vi "ModbusRxLoop.vi"(11 "ModbusPortSettings":T1={"TxPort"="ModbusPort1Tx", "TxDataFIFO"="ModbusPort1TxFIFO", "TxInternalDataFIFO"="ModbusPort1TxInternalFIFO", "TxHealthAndStatusFIFO"="ModbusPort1TxHealthAndStatusFIFO", "RxPort"="ModbusPort1Rx", "RxDataFIFO"="ModbusPort1RxFIFO", "RxHealthAndStatusFIFO"="ModbusPort1RxHealthAndStatusFIFO", "WaitForRxFrameRegister"="ModbusPort1WaitForRxControl", "BaseHealthAndStatusAddress"=0, "IRQAddress"=0, "TriggerIRQRegister"="ModbusPort1IRQControl", "SoftwareControlledTrigger"="ModbusSoftwareControlledTrigger", "TimestampRegister"="TimestampRegister", "TxTimestampFIFO"="ModbusPort1TimestampFIFO"}) -> ()   [LabVIEW 2016, in "FPGAModbus.lvlib"]
uses:
  FPGAModbus.lvlib
  DataTypes/ModbusPortSettings.ctl
  DataTypes/ModbusRxLoopData.ctl
  DataTypes/ModbusRxStates.ctl
  <vilib>/Platform/TimedLoop/XDataNode/timing_clust.ctl
  <vilib>/Platform/TimedLoop/XDataNode/nitl_modes.ctl
  <vilib>/Platform/TimedLoop/XDataNode/wakeup.ctl
  Common_FPGA_HealthAndStatus/DataTypes/HealthAndStatusUpdateMode.ctl
  <vilib>/rvi/Emulation/niFpgaSctlEmulationGetInTimedLoop.vi
  <vilib>/rvi/Emulation/niFpgaEmulationReportErrorSimple.vi
  <vilib>/rvi/Emulation/niFpgaGetClockAttributes.vi
  <vilib>/rvi/Emulation/niFpgaCriticalErrorInLSC.vi
  <vilib>/rvi/DataTransferAndStorage/Container/Common/niFpgaContainerExecOnDevCompGetState.vi
  <vilib>/rvi/Emulation/niFpgaEmulationIsFPGAContextNoSignature.vi
  <vilib>/rvi/DataTransferAndStorage/Container/Common/niFpgaContainerGetUniqueNameForEmu.vi
  <vilib>/rvi/Memory/Memory_Emulation/niFpgaMemoryEmulationCacheClearOnFirstRun.vi
  <vilib>/rvi/Memory/Memory_Emulation/nirvimemoryEmulationManagerCache_MakeExclusive.vi
  <vilib>/rvi/Memory/Memory_Emulation/niFpgaMemoryEmulationValidateCache.vi
  <vilib>/rvi/Memory/Memory_Emulation/nirvimemoryEmulationManagerCache_InsertValue.vi
  <vilib>/Utility/error.llb/Clear Errors.vi
  <vilib>/rvi/Memory/Memory_Emulation/nirvimemoryEmulationManagerCache_ReleaseExclusive.vi
  <vilib>/rvi/Memory/Memory_Emulation/nirvimemoryEmulationManagerCache_GetValue.vi
  <vilib>/rvi/Memory/Memory_Emulation/nirvimemoryEmulationManagerCache_SetValue.vi
  <vilib>/rvi/Emulation/niFpgaProcessEmulError.vi
  <vilib>/rvi/eio/common/nirviEmuTemplateMethod_errors.vi
  <vilib>/rvi/errors/niFpgaSetErrorForExecOnDevCompSimple.vi
  <vilib>/rvi/eio/common/nirviEmuReportErrorAndStop.vi
  <vilib>/rvi/FIFO/Fifo_Resource/nirvififoEmulationSetSize.vi
  <vilib>/rvi/FIFO/Fifo_Resource/nirviFifoEmulationQueueMgr.vi
  <instcachedir>/0/nirviFifoEmulationQueueMgr_E5CAEC123FF24DC58D834DCA3CDAA9B5.lvgen/nirviFifoEmulationQueueMgr_E5CAEC123FF24DC58D834DCA3CDAA9B5_002.vi
  <vilib>/rvi/FIFO/Fifo_Resource/nirvififoEmulationDetermineInputValidOut.vi
  <vilib>/rvi/FIFO/Fifo_Resource/nirvififoEmulationCreateLock.vi
  <vilib>/rvi/FIFO/Fifo_Resource/nirvififoEmulationObtainLock.vi
  <vilib>/rvi/FIFO/Fifo_Resource/nirvififoEmulationReleaseLock.vi
  <vilib>/rvi/occurrence/nirviWaitOnOccurrenceBase.vi
  <vilib>/rvi/errors/nirviReportUnexpectedCaseInternalError.vi
  <vilib>/rvi/errors/nirviReportUnexpectedCaseInternalError (U32).vi
  <vilib>/rvi/interface/RandomDataEmulation/niFpgaRandomDataHandleErrors.vi
  <vilib>/Platform/TimedLoop/XDataNode/XDataNode.xnode
  <vilib>/rvi/DataTransferAndStorage/Container/XNode/niFpgaContainer.xnode
  <vilib>/rvi/DataTransferAndStorage/Register/Emulation/niFpgaRegisterEmulationRefIn.vi
  <vilib>/eio/EIONode/EIONode.xnode
  <vilib>/rvi/FIFO/Fifo_Resource/niFpgaFifoEmulationRefIn.vi
  Common_FPGA_HealthAndStatus/FPGAHealthAndStatus.lvlib
  <vilib>/Platform/TimedLoop/XDataNode/XDNodeRunTimeDep.lvlib
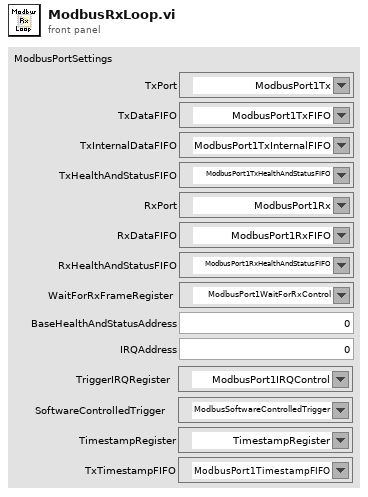
[diagram p1: front panel]
types:
  T1 = typedef "FPGAModbus.lvlib/ModbusPortSettings.ctl" = cluster{"TxPort":refnum<k21>, "TxDataFIFO":refnum<k21>, "TxInternalDataFIFO":refnum<k21>, "TxHealthAndStatusFIFO":refnum<k21>, "RxPort":refnum<k21>, "RxDataFIFO":refnum<k21>, "RxHealthAndStatusFIFO":refnum<k21>, "WaitForRxFrameRegister":refnum<k21>, "BaseHealthAndStatusAddress":u32, "IRQAddress":u8, "TriggerIRQRegister":refnum<k21>, "SoftwareControlledTrigger":refnum<k21>, "TimestampRegister":refnum<k21>, "TxTimestampFIFO":refnum<k21>}
  T2 = typedef "FPGAModbus.lvlib/ModbusRxLoopData.ctl" = cluster{"State":T3, "DelayTicks":u16, "StateAfterDelay":T3, "NumberOfSamples":u16, "Sample":u8, "Data":u16, "Bits":u16, "StateAfterInsertSample":T3, "ReceivedData":bool, "EnqueueDataTime":u32, "PreviousLevel":bool, "Timestamp":u64, "TimestampWord":u8}
  T3 = typedef "FPGAModbus.lvlib/ModbusRxStates.ctl" = enum16{"WaitForFallingEdge", "Delay", "SampleStartBit", "SampleBit", "EnqueueData", "EnqueueEndOfFrame", "EnqueueTimestamp"}
  T4 = typedef "XDNodeRunTimeDep.lvlib/timing_clust.ctl" = cluster{"Expected End [f-1]":u64, "Actual End [f-1]":u64, "Finished Late? [f-1]":bool, "Expected End [i-1]":u64, "Actual End [i-1]":u64, "Finished Late? [i-1]":bool, "Expected Start [i]":u64, "Actual Start [i]":u64, "Expected Start [f]":u64, "Actual Start [f]":u64, "Source Name":string, "Structure Name":string, "Period":i64, "Deadline":i64, "Offset":i64, "Start":i64, "Priority":i32, "Timeout":i32, "Mode":T5, "Wakeup Reason":T6, "Error":errorcluster, "Source Type":string, "Secondary Source Type":string, "Global End Time":u64, "Global Start Time":u64, "Frame Duration":u64, "Iteration Duration":u64, "Assigned CPU":i32, "I/O Scan Engine Mode":u32}
  T5 = typedef "XDNodeRunTimeDep.lvlib/nitl_modes.ctl" = enum32{"No Change", "Process missed periods, maintain original phase", "Discard missed periods, maintain original phase", "Process missed periods, ignore original phase", "Discard missed periods, ignore original phase"}
  T6 = typedef "XDNodeRunTimeDep.lvlib/wakeup.ctl" = enum32{"Normal", "Aborted", "Asynchronous wakeup", "Timing source error", "Timed loop error", "Timeout"}
  T7 = typedef "FPGAHealthAndStatus.lvlib/HealthAndStatusUpdateMode.ctl" = enum8{"NOP", "Set", "Add", "Subtract", "Or"}
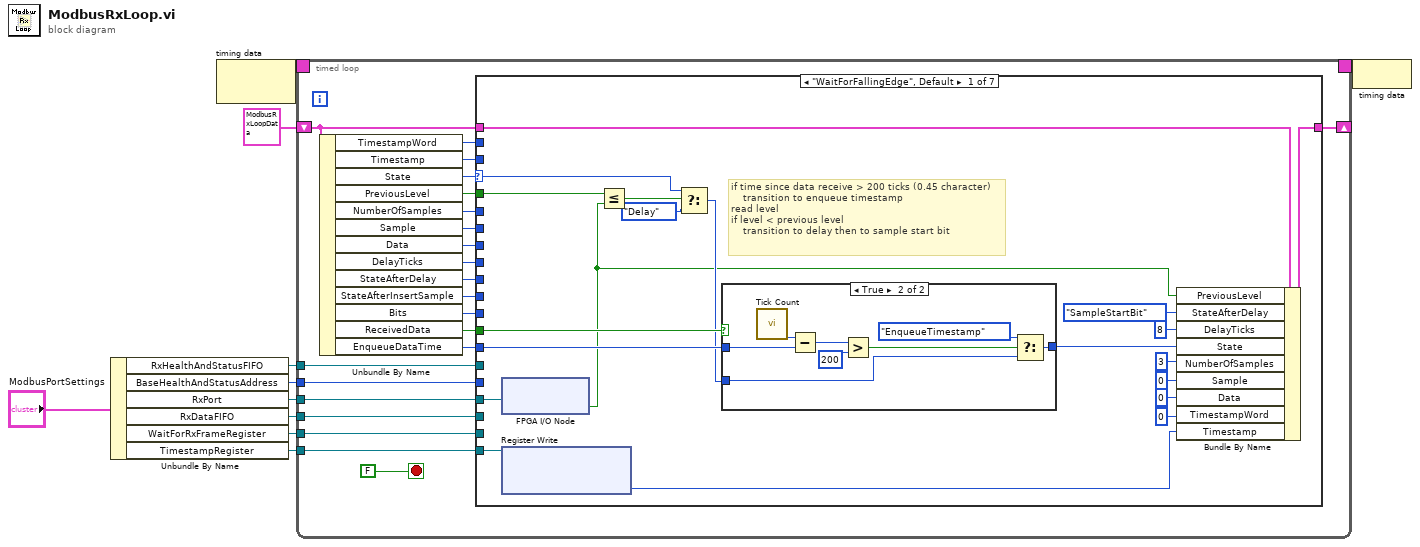
[diagram p0: block diagram]
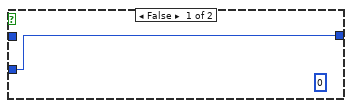
[diagram p2: hidden frame]
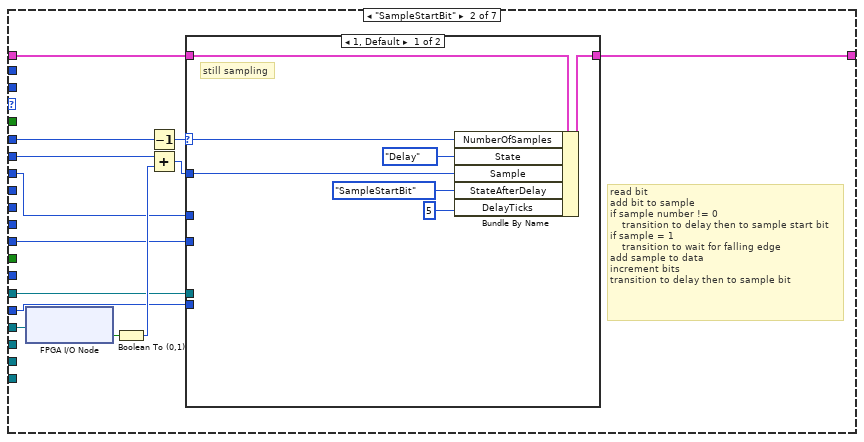
[diagram p3: hidden frame]
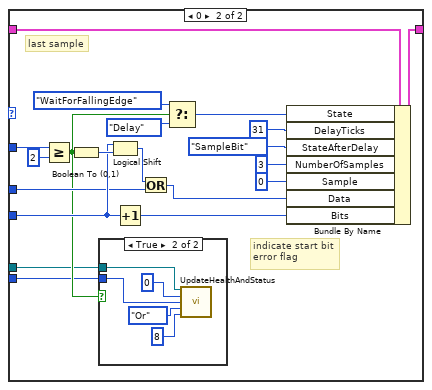
[diagram p4: hidden frame]
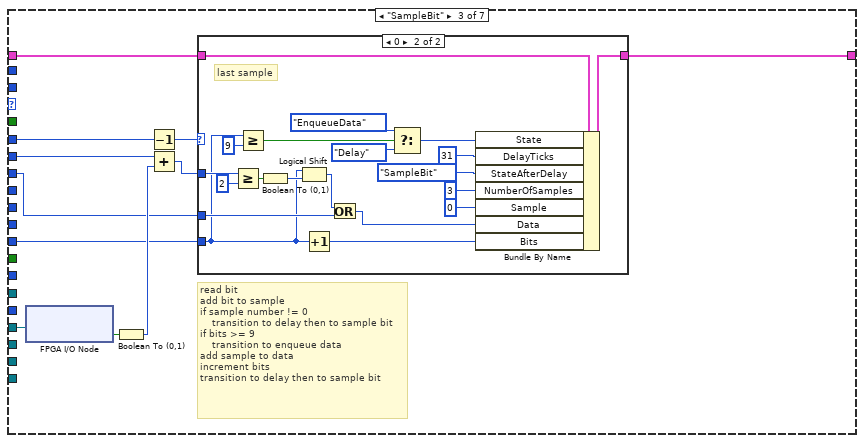
[diagram p6: hidden frame]
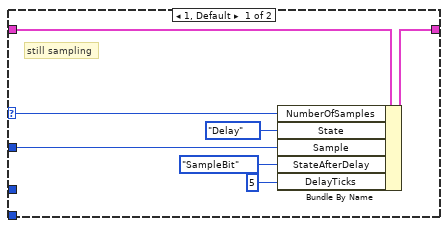
[diagram p7: hidden frame]
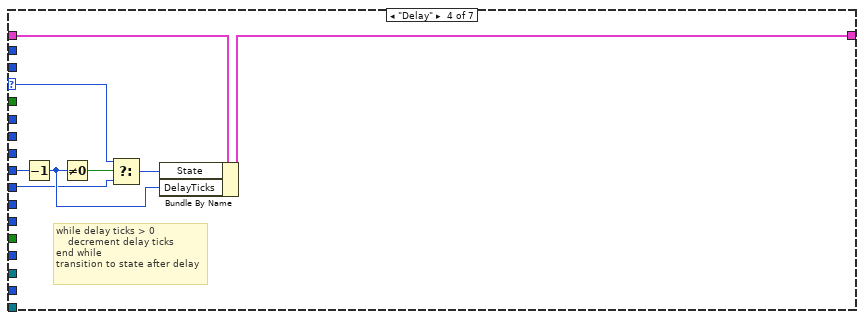
[diagram p8: hidden frame]
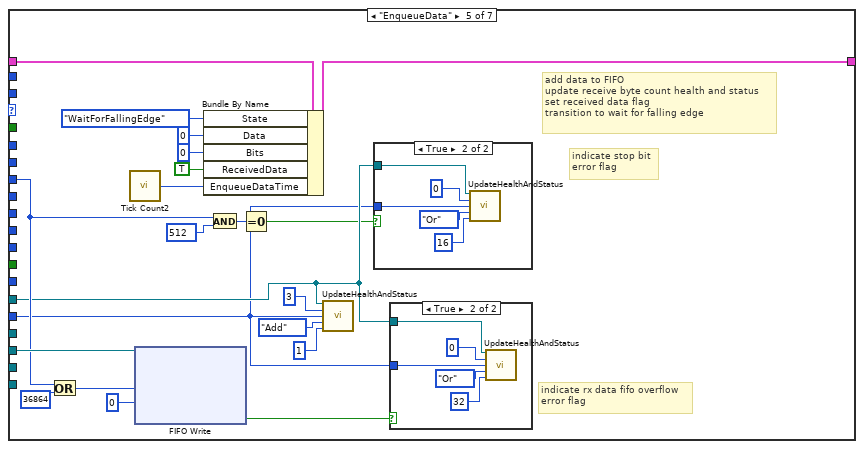
[diagram p9: hidden frame]
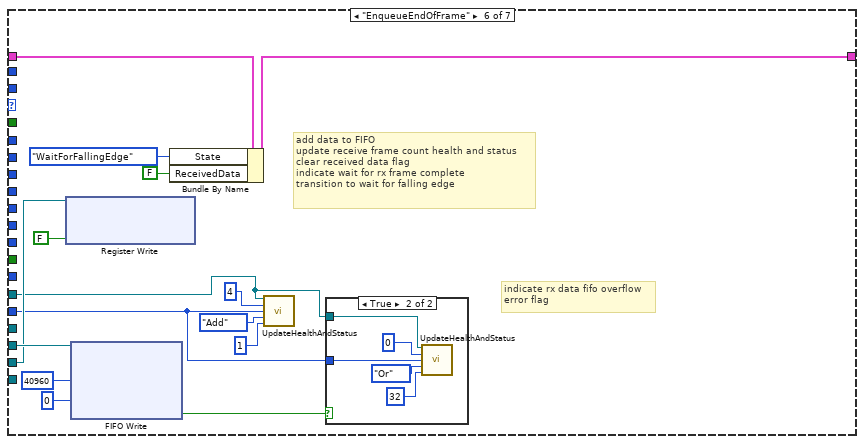
[diagram p12: hidden frame]
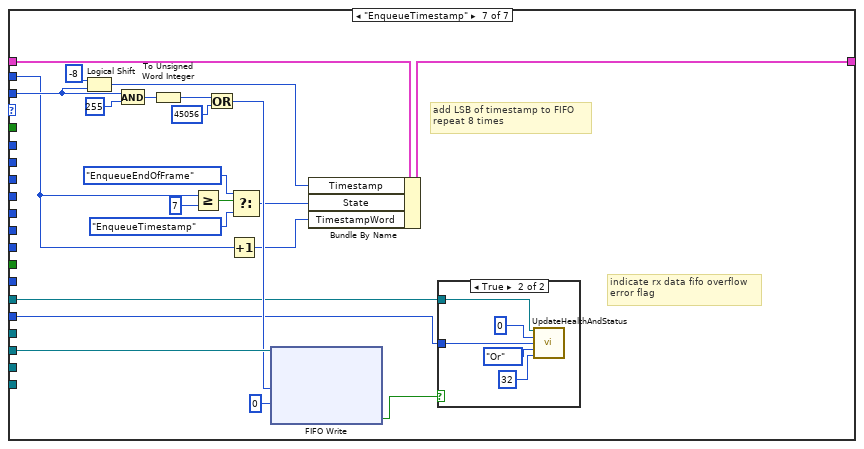
[diagram p14: hidden frame]
diagram:
  n1 = Unbundle By Name("ModbusPortSettings") -> ("RxHealthAndStatusFIFO"=w7:refnum<k21>, "BaseHealthAndStatusAddress"=w4:u32, "RxPort"=w5:refnum<k21>, "RxDataFIFO"=w6:refnum<k21>, "WaitForRxFrameRegister"=w8:refnum<k21>, "TimestampRegister"=w1:refnum<k21>)
  n2 = node-c288() -> (w10:T4)  [unwired: 1 in]
  n3 = timed-loop {
    tunnel: w5 -> [w30]
    tunnel: w6 -> [w21]
    shift-right: [w29] -> _
    shift-left: T2 {"State"=enum."WaitForFallingEdge", "DelayTicks"=0, "StateAfterDelay"=enum."WaitForFallingEdge", "NumberOfSamples"=0, "Sample"=0, "Data"=0, "Bits"=0, "StateAfterInsertSample"=enum."WaitForFallingEdge", "ReceivedData"=FALSE, "EnqueueDataTime"=0, "PreviousLevel"=FALSE, "Timestamp"=0, "TimestampWord"=0} ("ModbusRxLoop") -> [w32]
    tunnel: w4 -> [w18]
    timing: w10 -> [_]
    timing-out: [_] -> w9
    tunnel: w7 -> [w16]
    tunnel: w8 -> [w15]
    tunnel: w1 -> [w13]
    stop <- FALSE stop-if-true
    n4 = Unbundle By Name(w32) -> ("TimestampWord"=w11:u8, "Timestamp"=w12:u64, "State"=w31:T3, "PreviousLevel"=w17:bool, "NumberOfSamples"=w28:u16, "Sample"=w27:u8, "Data"=w26:u16, "DelayTicks"=w25:u16, "StateAfterDelay"=w24:T3, "StateAfterInsertSample"=w23:T3, "Bits"=w22:u16, "ReceivedData"=w19:bool, "EnqueueDataTime"=w20:u32)
    n5 = case shown="\"WaitForFallingEdge\", Default" w31 {
      selector: w31 -> [w51 _ _ w149 _ _ _]
      tunnel: w32 -> [w45 w69 w112 w146 w172 w195 w225]
      tunnel: w30 -> [w52 w73 w116 _ _ _ _]
      tunnel: [w48 w68 w111 w145 w171 w192 w224] -> w29
      tunnel: w28 -> [_ w74 w117 _ _ _ _]
      tunnel: w27 -> [_ w71 w114 _ _ _ _]
      tunnel: w26 -> [_ w64 w107 _ w158 _ _]
      tunnel: w25 -> [_ _ _ w147 _ _ _]
      tunnel: w24 -> [_ _ _ w148 _ _ _]
      tunnel: w23 -> [_ _ _ _ _ _ _]
      tunnel: w22 -> [_ w65 w108 _ _ _ _]
      tunnel: w21 -> [_ _ _ _ w173 w198 w216]
      tunnel: w20 -> [w50 _ _ _ _ _ _]
      tunnel: w19 -> [w49 _ _ _ _ _ _]
      tunnel: w18 -> [_ w62 _ _ w154 w186 w211]
      tunnel: w17 -> [w39 _ _ _ _ _ _]
      tunnel: w16 -> [_ w63 _ _ w155 w185 w213]
      tunnel: w15 -> [_ _ _ _ _ w187 _]
      tunnel: w13 -> [w35 _ _ _ _ _ _]
      tunnel: w12 -> [_ _ _ _ _ _ w209]
      tunnel: w11 -> [_ _ _ _ _ _ w205]
      frame "WaitForFallingEdge", Default {
        # "if time since data receive > 200 ticks (0.45 character)\n    transition to enqueue timestamp\nread level\nif level < previous level\n    transition to delay then to sample start bit"
        n6 = xnode "FPGA I/O Node"("FPGA I/O In"=w52) -> ("I/O Item"=w36:bool)  [unwired: 1 out]
        n7 = xnode "Register Write"("Register In"=w35) -> ("Data"=w34:u64)  [unwired: 1 out]
        n8 = Less Or Equal?(x=w39, y=w36) -> (x <= y?=w42:bool)
        n9 = Select(t=w51, s=w42, f=ModbusRxStates."Delay" ("State After Delay")) -> (s? t:f=w41:T3)
        n10 = case shown="True" w49 {
          tunnel: w50 -> [_ w60]
          tunnel: w41 -> [w53 w55]
          tunnel: [w53 w54] -> w46
          frame False {
            (unwired) u16 0
          }
          frame True {
            n11 = call "Tick Count"() -> ("Tick Count(Ticks)"=w61:u32)
            n12 = Subtract(x=w61, y=w60) -> (x-y=w59:u32)
            n13 = Greater?(x=w59, y=u32 200) -> (0:w57:bool)
            n14 = Select(t=ModbusRxStates."EnqueueTimestamp" ("f"), s=w57, f=w55) -> (s? t:f=w54:T3)
          }
        }
        n15 = Bundle By Name(cluster=w45, "PreviousLevel"=w36, "StateAfterDelay"=ModbusRxStates."SampleStartBit" ("State After Delay"), "DelayTicks"=u16 8 ("Sample"), "State"=w46, "NumberOfSamples"=u16 3 ("Number of Samples"), "Sample"=u8 0, "Data"=u16 0, "TimestampWord"=u8 0, "Timestamp"=w34) -> (w48:T2)
      }
      frame "SampleStartBit" {
        # "read bit\nadd bit to sample\nif sample number != 0\n    transition to delay then to sample start bit\nif sample = 1\n    transition to wait for falling edge\nadd sample to data\nincrement bits\ntransition to delay then to sample bit"
        n16 = xnode "FPGA I/O Node"("FPGA I/O In"=w73) -> ("I/O Item"=w72:bool)  [unwired: 1 out]
        n17 = Boolean To (0,1)(Boolean=w72) -> (0, 1=w70:i16)
        n18 = Decrement(x=w74) -> (x-1=w66:u16)
        n19 = Add(x=w71, y=w70) -> (x+y=w67:i16)
        n20 = case shown="1, Default" w66 {
          selector: w66 -> [w78 _]
          tunnel: w67 -> [w79 w99]
          tunnel: w69 -> [w81 w101]
          tunnel: [w80 w100] -> w68
          tunnel: w65 -> [_ w95]
          tunnel: w64 -> [_ w94]
          tunnel: w63 -> [_ w83]
          tunnel: w62 -> [_ w82]
          frame 1, Default {
            # "still sampling"
            n21 = Bundle By Name(cluster=w81, "NumberOfSamples"=w78, "State"=ModbusRxStates."Delay" ("State After Action"), "Sample"=w79, "StateAfterDelay"=ModbusRxStates."SampleStartBit" ("State After Delay"), "DelayTicks"=u16 5 ("Delay Ticks")) -> (w80:T2)
          }
          frame 0 {
            # "indicate start bit\nerror flag"
            # "last sample"
            n22 = Greater Or Equal?(x=w99, y=i16 2) -> (x >= y?=w84:bool)
            n23 = Boolean To (0,1)(Boolean=w84) -> (0, 1=w96:i16)
            n24 = case shown="True" w84 {
              tunnel: w83 -> [_ w103]
              tunnel: w82 -> [_ w102]
              frame False {
              }
              frame True {
                n25 = call "UpdateHealthAndStatus.vi"("InternalHealthAndStatusFIFO"=w103, "AddressOffset"=u32 0 ("x"), "BaseAddress"=w102, "HealthAndStatusUpdateMode"=HealthAndStatusUpdateMode."Or" ("Telemetry Update Mode"), "Data"=u32 8) -> ()  [unwired: 11 in]
              }
            }
            n26 = Logical Shift(y=w95, x=w96) -> (x << y=w97:i16)
            n27 = Increment(x=w95) -> (x+1=w93:u16)
            n28 = Or(x=w97, y=w94) -> (x .or. y?=w92:u16)
            n29 = Select(t=ModbusRxStates."WaitForFallingEdge", s=w84, f=ModbusRxStates."Delay" ("State After Action")) -> (s? t:f=w85:T3)
            n30 = Bundle By Name(cluster=w101, "State"=w85, "DelayTicks"=u16 31 ("Delay Ticks"), "StateAfterDelay"=ModbusRxStates."SampleBit" ("State After Delay"), "NumberOfSamples"=u16 3 ("Number of Samples"), "Sample"=u8 0, "Data"=w92, "Bits"=w93) -> (w100:T2)
          }
        }
      }
      frame "SampleBit" {
        # "read bit\nadd bit to sample\nif sample number != 0\n    transition to delay then to sample bit\nif bits >= 9\n    transition to enqueue data\nadd sample to data\nincrement bits\ntransition to delay then to sample bit"
        n31 = xnode "FPGA I/O Node"("FPGA I/O In"=w116) -> ("I/O Item"=w115:bool)  [unwired: 1 out]
        n32 = Boolean To (0,1)(Boolean=w115) -> (0, 1=w113:i16)
        n33 = Decrement(x=w117) -> (x-1=w109:u16)
        n34 = Add(x=w114, y=w113) -> (x+y=w110:i16)
        n35 = case shown="0" w109 {
          selector: w109 -> [w121 _]
          tunnel: w110 -> [w122 w142]
          tunnel: w112 -> [w124 w144]
          tunnel: [w123 w143] -> w111
          tunnel: w108 -> [_ w125]
          tunnel: w107 -> [_ w138]
          frame 1, Default {
            # "still sampling"
            n36 = Bundle By Name(cluster=w124, "NumberOfSamples"=w121, "State"=ModbusRxStates."Delay" ("State After Action"), "Sample"=w122, "StateAfterDelay"=ModbusRxStates."SampleBit" ("State After Delay"), "DelayTicks"=u16 5 ("Delay Ticks")) -> (w123:T2)
          }
          frame 0 {
            # "last sample"
            n37 = Greater Or Equal?(x=w142, y=i16 2) -> (x >= y?=w133:bool)
            n38 = Greater Or Equal?(x=w125, y=u16 9) -> (x >= y?=w126:bool)
            n39 = Boolean To (0,1)(Boolean=w133) -> (0, 1=w139:i16)
            n40 = Logical Shift(y=w125, x=w139) -> (x << y=w140:i16)
            n41 = Increment(x=w125) -> (x+1=w137:u16)
            n42 = Or(x=w140, y=w138) -> (x .or. y?=w136:u16)
            n43 = Select(t=ModbusRxStates."EnqueueData", s=w126, f=ModbusRxStates."Delay" ("State After Action")) -> (s? t:f=w128:T3)
            n44 = Bundle By Name(cluster=w144, "State"=w128, "DelayTicks"=u16 31 ("Delay Ticks"), "StateAfterDelay"=ModbusRxStates."SampleBit" ("State After Delay"), "NumberOfSamples"=u16 3 ("Number of Samples"), "Sample"=u8 0, "Data"=w136, "Bits"=w137) -> (w143:T2)
          }
        }
      }
      frame "Delay" {
        # "while delay ticks > 0\n    decrement delay ticks\nend while\ntransition to state after delay"
        n45 = Decrement(x=w147) -> (x-1=w150:u16)
        n46 = Not Equal To 0?(x=w150) -> (x != 0?=w152:bool)
        n47 = Select(t=w149, s=w152, f=w148) -> (s? t:f=w151:T3)
        n48 = Bundle By Name(cluster=w146, "State"=w151, "DelayTicks"=w150) -> (w145:T2)
      }
      frame "EnqueueData" {
        # "indicate stop bit\nerror flag"
        # "indicate rx data fifo overflow\nerror flag"
        # "add data to FIFO\nupdate receive byte count health and status\nset received data flag\ntransition to wait for falling edge"
        n49 = Or(x=w158, y=u16 36864 ("Data")) -> (x .or. y?=w164:u16)
        n50 = call "Tick Count2"() -> ("Tick Count(Ticks)"=w168:u32)
        n51 = xnode ("FIFO Write")("Element"=w164, "Timeout"=0, "FIFO In"=w173) -> ("Timed Out?"=w159:bool)  [unwired: 1 out]
        n52 = Bundle By Name(cluster=w172, "State"=ModbusRxStates."WaitForFallingEdge", "Data"=u16 0, "Bits"=u16 0, "ReceivedData"=TRUE ("Received Data"), "EnqueueDataTime"=w168) -> (w171:T2)
        n53 = And(x=w158, y=u16 512 ("Data")) -> (x .and. y?=w156:u16)
        n54 = Equal To 0?(x=w156) -> (x = 0?=w153:bool)
        n55 = call "UpdateHealthAndStatus.vi"("InternalHealthAndStatusFIFO"=w155, "AddressOffset"=u32 3 ("x"), "BaseAddress"=w154, "HealthAndStatusUpdateMode"=HealthAndStatusUpdateMode."Add" ("Telemetry Update Mode"), "Data"=u64 1) -> ()  [unwired: 11 in]
        n56 = case shown="True" w153 {
          tunnel: w155 -> [_ w175]
          tunnel: w154 -> [_ w174]
          frame False {
          }
          frame True {
            n57 = call "UpdateHealthAndStatus.vi"("InternalHealthAndStatusFIFO"=w175, "AddressOffset"=u32 0 ("x"), "BaseAddress"=w174, "HealthAndStatusUpdateMode"=HealthAndStatusUpdateMode."Or" ("Telemetry Update Mode"), "Data"=u64 16) -> ()  [unwired: 11 in]
          }
        }
        n58 = case shown="True" w159 {
          tunnel: w155 -> [_ w180]
          tunnel: w154 -> [_ w179]
          frame False {
          }
          frame True {
            n59 = call "UpdateHealthAndStatus.vi"("InternalHealthAndStatusFIFO"=w180, "AddressOffset"=u32 0 ("x"), "BaseAddress"=w179, "HealthAndStatusUpdateMode"=HealthAndStatusUpdateMode."Or" ("Telemetry Update Mode"), "Data"=u64 32) -> ()  [unwired: 11 in]
          }
        }
      }
      frame "EnqueueEndOfFrame" {
        # "indicate rx data fifo overflow\nerror flag"
        # "add data to FIFO\nupdate receive frame count health and status\nclear received data flag\nindicate wait for rx frame complete\ntransition to wait for falling edge"
        n60 = xnode ("Register Write")("Data"=FALSE, "Register In"=w187) -> ()  [unwired: 1 out]
        n61 = xnode ("FIFO Write")("Element"=u16 40960, "Timeout"=0, "FIFO In"=w198) -> ("Timed Out?"=w184:bool)  [unwired: 1 out]
        n62 = Bundle By Name(cluster=w195, "State"=ModbusRxStates."WaitForFallingEdge", "ReceivedData"=FALSE ("Received Data")) -> (w192:T2)
        n63 = call "UpdateHealthAndStatus.vi"("InternalHealthAndStatusFIFO"=w185, "AddressOffset"=u32 4 ("x"), "BaseAddress"=w186, "HealthAndStatusUpdateMode"=HealthAndStatusUpdateMode."Add" ("Telemetry Update Mode"), "Data"=u64 1) -> ()  [unwired: 11 in]
        n64 = case shown="True" w184 {
          tunnel: w185 -> [_ w200]
          tunnel: w186 -> [_ w199]
          frame False {
          }
          frame True {
            n65 = call "UpdateHealthAndStatus.vi"("InternalHealthAndStatusFIFO"=w200, "AddressOffset"=u32 0 ("x"), "BaseAddress"=w199, "HealthAndStatusUpdateMode"=HealthAndStatusUpdateMode."Or" ("Telemetry Update Mode"), "Data"=u64 32) -> ()  [unwired: 11 in]
          }
        }
      }
      frame "EnqueueTimestamp" {
        # "indicate rx data fifo overflow\nerror flag"
        # "add LSB of timestamp to FIFO\nrepeat 8 times"
        n66 = Logical Shift(y=i16 -8, x=w209) -> (x << y=w207:u64)
        n67 = And(x=w209, y=u64 255) -> (x .and. y?=w219:u64)
        n68 = To Unsigned Word Integer(number=w219) -> (unsigned 16bit integer=w217:u16)
        n69 = Greater Or Equal?(x=w205, y=u8 7) -> (x >= y?=w223:bool)
        n70 = Or(x=w217, y=u16 45056) -> (x .or. y?=w214:u16)
        n71 = Increment(x=w205) -> (x+1=w206:u8)
        n72 = Select(t=ModbusRxStates."EnqueueEndOfFrame" ("State"), s=w223, f=ModbusRxStates."EnqueueTimestamp") -> (s? t:f=w210:T3)
        n73 = xnode ("FIFO Write")("Element"=w214, "Timeout"=0, "FIFO In"=w216) -> ("Timed Out?"=w212:bool)  [unwired: 1 out]
        n74 = Bundle By Name(cluster=w225, "Timestamp"=w207, "State"=w210, "TimestampWord"=w206) -> (w224:T2)
        n75 = case shown="True" w212 {
          tunnel: w213 -> [_ w227]
          tunnel: w211 -> [_ w226]
          frame False {
          }
          frame True {
            n76 = call "UpdateHealthAndStatus.vi"("InternalHealthAndStatusFIFO"=w227, "AddressOffset"=u32 0 ("x"), "BaseAddress"=w226, "HealthAndStatusUpdateMode"=HealthAndStatusUpdateMode."Or" ("Telemetry Update Mode"), "Data"=u64 32) -> ()  [unwired: 11 in]
          }
        }
      }
    }
  }
  n77 = node-c288(w9) -> ()
